vi "Actor Core.vi"(8 "error in":errorcluster, 11 "Car Wash Status View Definition In":refnum<class "Car Wash Status View Definition.lvclass">) -> (0 "error out":errorcluster, 3 "Actor out":refnum<class "Actor.lvclass">)   [LabVIEW 2019, in "Car Wash Status View Definition.lvclass"]
doc: "(<B>Filename</B>: Actor Framework.lvlib:Actor.lvclass:Actor Core.vi)\n\nReceives messages to the actor, reacts to them, and initiates any error handling that may shut the actor down.\n\nDescendant classes may override this VI to append parallel tasks for the actor to complete while it handles messages. Overrides use the Call Parent Method node.\n\n<License>\nCopyright © 2017 Composed Systems, LLC | All rights reserved\nwww.composed.io\n\nAuthor: Ethan Stern <ethan.stern@composed.io>\n\nThis software is provided \"AS IS\" WITHOUT WARRANTIES, either express or implied, AND IS FOR EDUCATIONAL PURPOSES ONLY.\n</License>"
uses:
  <vilib>/gpm_packages/@cs/Car-wash/Source/Car Wash Status View Definition/Car Wash Status View Definition/Car Wash Status View Definition.lvclass
  C:/Program Files/National Instruments/LabVIEW 2019/vi.lib/gpm_packages/@cs/mva-viewable/Source/IViewable/IViewable/IViewable.lvclass
  <vilib>/ActorFramework/Actor/Actor.lvclass
  <vilib>/gpm_packages/@cs/Car-wash/Source/Car Wash Status View Definition/Car Wash Status View Definition/Car Wash Status View Definition.lvclass/Car Wash Status View Definition.ctl
  <vilib>/gpm_packages/@cs/mva-viewable/Source/IViewable/IViewable/IViewable.lvclass
panel:
  # "This is a definition view"
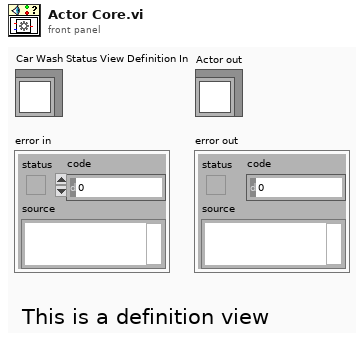
[diagram p1: front panel]
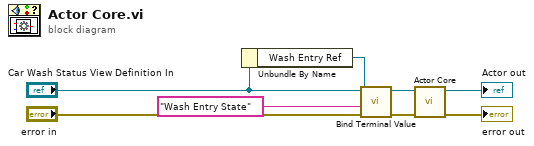
[diagram p0: block diagram]
diagram:
  n1 = Unbundle By Name("Car Wash Status View Definition In") -> ("Wash Entry Ref"=w2:refnum<vi>)
  n2 = call <vilib>:"Bind Terminal Value.vi"("error in (no error)"="error in", "Datum Name (\"\"=Use Control Label)"="Wash Entry State" ("Datum Name (\"\"=Use Control Label)"), "Ctl Refnum"=w2, "IViewable in"="Car Wash Status View Definition In") -> ("error out"=w3:errorcluster, "IViewable out"=w4:refnum<class "Car Wash Status View Definition.lvclass">)  [unwired: 6 in]
  n3 = call-parent "Actor Core.vi"("error in"=w3, "IViewable In"=w4) -> ("error out"=→"error out":errorcluster, "Actor out"=→"Actor out":refnum<class "Actor.lvclass">)  [unwired: 8 in]
